vi "Panel.vi"() -> ()   [LabVIEW 2011]
uses:
  Global.vi
panel:
  in  "stop":bool
  out "Thermometer":dbl(slide) scale=0.0..50.0
  out "Tank":dbl(slide) scale=0.0..100.0
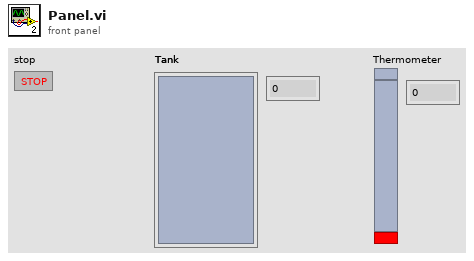
[diagram p1: front panel]
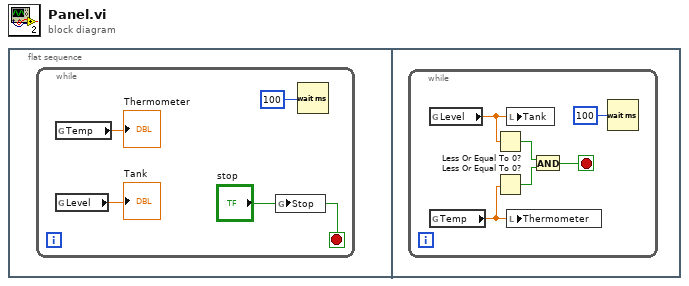
[diagram p0: block diagram]
diagram:
  n1 = flat-sequence {
    frame #0 {
      n2 = while {
        stop <- "stop" stop-if-true
        n3 = global read "Global.vi" "Temp"() -> (→"Thermometer":dbl)
        n4 = global read "Global.vi" "Level"() -> (→"Tank":dbl)
        n5 = global write "Global.vi" "Stop"("stop") -> ()
        n6 = Wait (ms)(milliseconds to wait=100) -> ()  [unwired: 1 out]
      }
    }
    frame #1 {
      n7 = while {
        stop <- w5 stop-if-true
        n8 = global read "Global.vi" "Level"() -> (w9:dbl)
        n9 = global read "Global.vi" "Temp"() -> (w8:dbl)
        n10 = Less Or Equal To 0?(x=w9) -> (x <= 0?=w7:bool)
        n11 = Less Or Equal To 0?(x=w8) -> (x <= 0?=w6:bool)
        n12 = local write "Tank"(w9) -> ()
        n13 = local write "Thermometer"(w8) -> ()
        n14 = And(x=w7, y=w6) -> (x .and. y?=w5:bool)
        n15 = Wait (ms)(milliseconds to wait=100) -> ()  [unwired: 1 out]
      }
    }
  }
